vi "HSFW Engine.vi"(0 "Notifier Name":string="Not a Name", 11 "HSFW Index":string[](array[string])) -> ()   [LabVIEW 2020]
uses:
  FW Type Defs/FW Notifier Type.ctl
  FW Type Defs/FW Actions.ctl
  C:/Users/Photonics03/Documents/Microscope-Control/Device Library/Filter Wheels/Edmund Optics/HSFW 84-889/OptecHID_FilterWheelAPI.dll
  OptecHID_FilterWheelAPI.dll
panel:
  out "Current Position":u8
  in  "Get Position":bool
  in  "FW Position":u8=1 min=1 max=8
  in  "Quit":bool
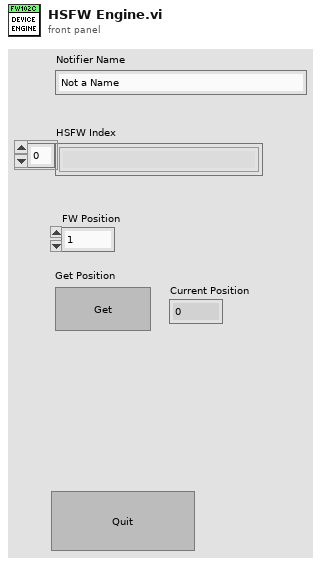
[diagram p1: front panel]
types:
  T1 = typedef "FW Actions.ctl" = enum16{"Set Position", "Get Position", "Get Num Positions", "Set Speed", "Confirm Pos", "Quit"}
  T2 = typedef "FW Notifier Type.ctl" = cluster{"Actions":T1, "Set Position":u8, "Actual Position":u8, "Speed":dbl, "Num Positions":u8, "Received":bool}
  T3 = enum32{"Invalid", "Standard", "Closed", "Hidden", "Minimized", "Maximized"}
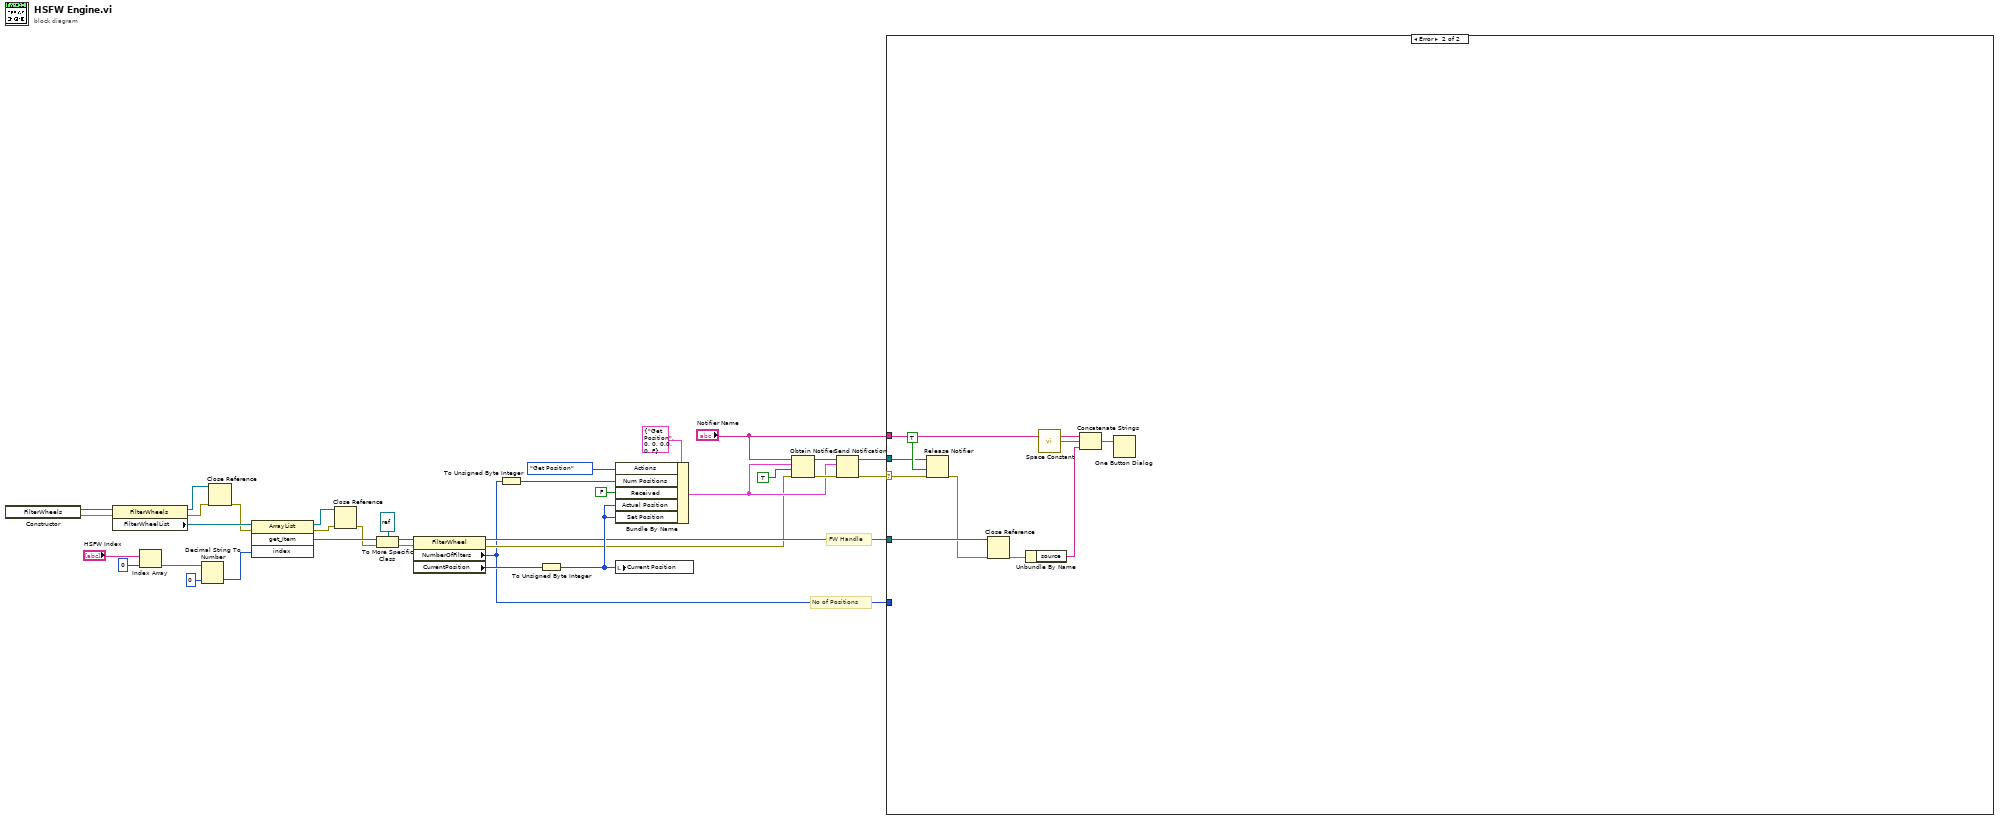
[diagram p0: block diagram]
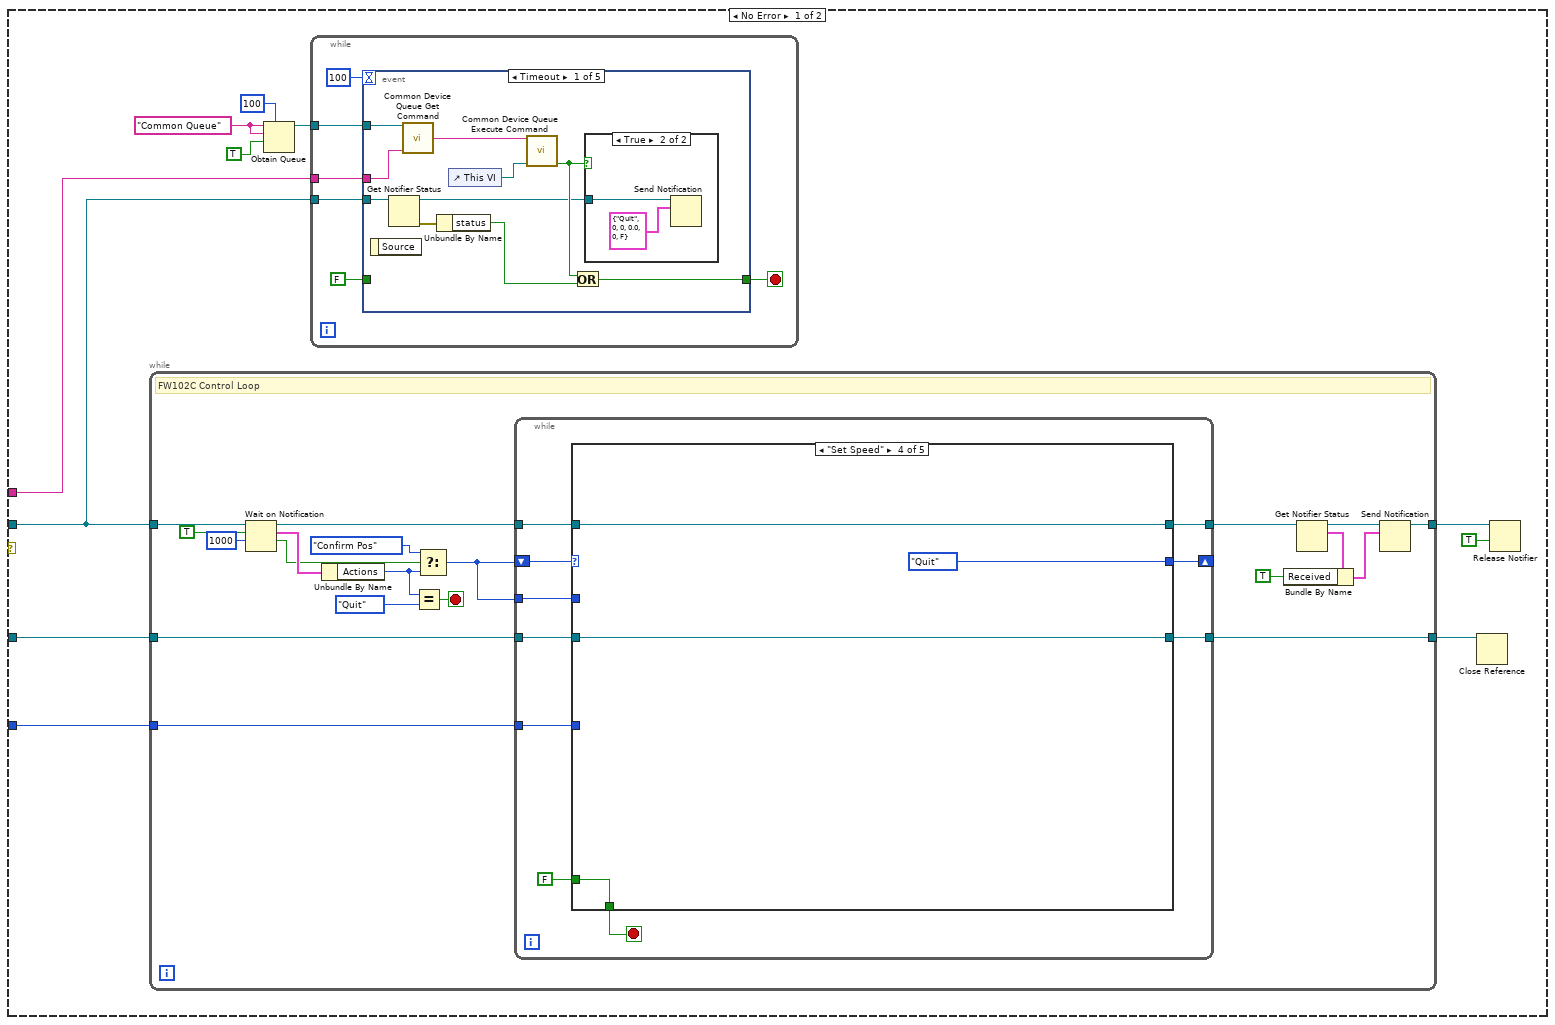
[diagram p2: hidden frame]
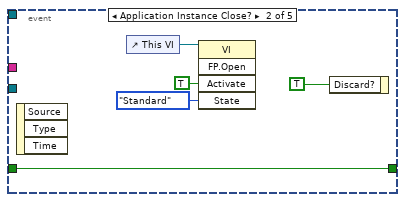
[diagram p4: hidden frame]
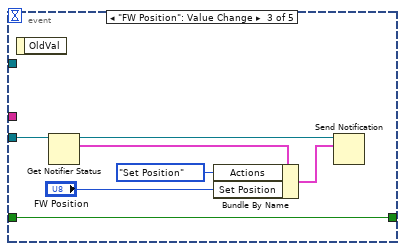
[diagram p5: hidden frame]
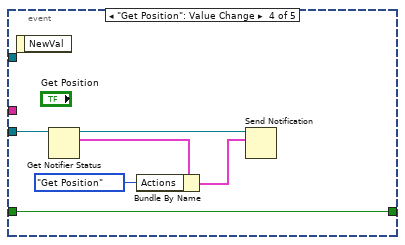
[diagram p6: hidden frame]
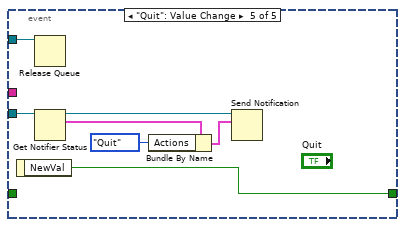
[diagram p7: hidden frame]
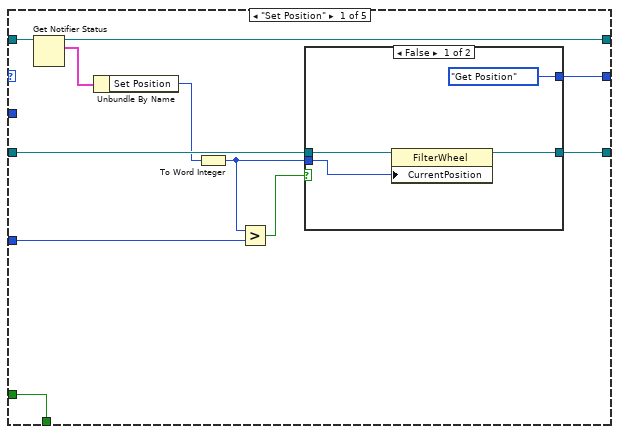
[diagram p8: hidden frame]
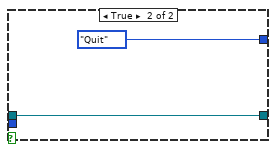
[diagram p9: hidden frame]
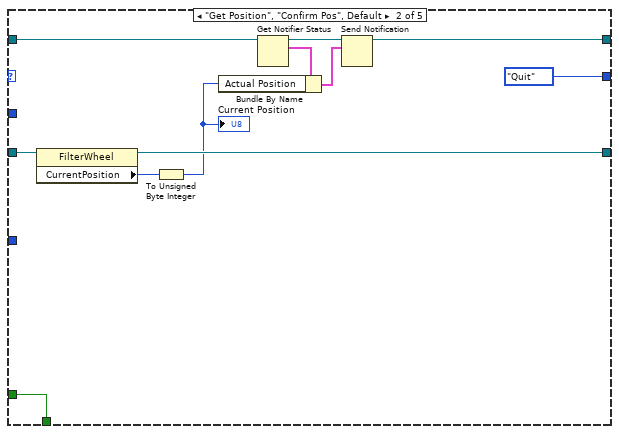
[diagram p10: hidden frame]
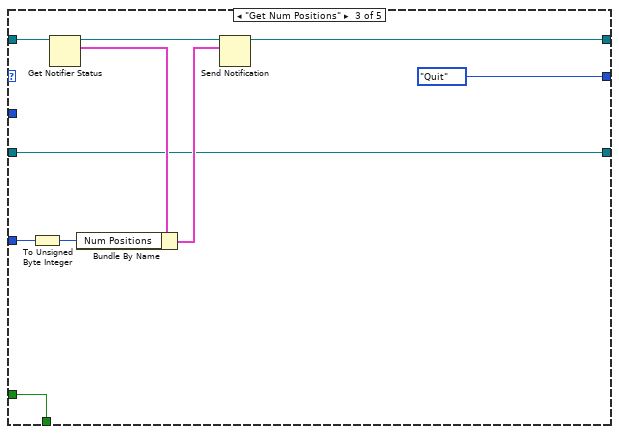
[diagram p11: hidden frame]
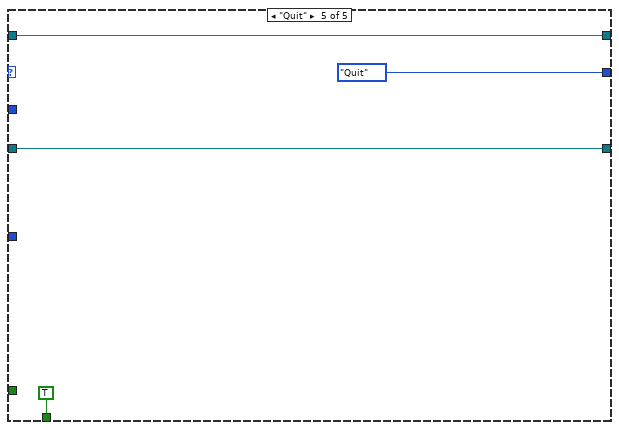
[diagram p12: hidden frame]
diagram:
  # "No of Positions"
  # "FW Handle"
  n1 = constructor class="FilterWheels"() -> (reference out=w20:refnum<k24>, error out=w17:errorcluster)  [unwired: 3 in, 1 out]
  n2 = property class="FilterWheels"(reference=w20, error in=w17) -> (reference out=w13:refnum<k24>, error out=w11:errorcluster, "FilterWheelList"=w21:refnum<k24>)
  n3 = Index Array(array="HSFW Index", index=0) -> (element=w16:string)
  n4 = Decimal String To Number(string=w16, default (0L)=0 ("default (0 I32)")) -> (number=w14:i32)  [unwired: 1 in, 1 out]
  n5 = Close Reference(reference=w13, error in (no error)=w11) -> (error out=w10:errorcluster)
  n6 = invoke class="ArrayList" method="get_Item"(reference=w21, error in=w10, "index"=w14) -> (reference out=w12:refnum<k24>, error out=w9:errorcluster, "get_Item"=w19:refnum<k24>)  [unwired: 1 in, 1 out]
  n7 = Close Reference(reference=w12, error in (no error)=w9) -> (error out=w8:errorcluster)
  n8 = To More Specific Class(target class=refnum<k24> refnum, reference=w19, error in=w8) -> (specific class reference=w7:refnum<k24>, error out=w4:errorcluster)
  n9 = property class="FilterWheel"(reference=w7, error in=w4) -> (reference out=w3:refnum<k24>, error out=w2:errorcluster, "NumberOfFilters"=w1:i16, "CurrentPosition"=w6:i16)
  n10 = To Unsigned Byte Integer(number=w1) -> (unsigned 8bit integer=w22:u8)
  n11 = To Unsigned Byte Integer(number=w6) -> (unsigned 8bit integer=w5:u8)
  n12 = Bundle By Name(cluster=T2 {"Actions"=enum."Get Position", "Set Position"=0, "Actual Position"=0, "Speed"=0.0, "Num Positions"=0, "Received"=FALSE} ("Note Type"), "Actions"=FW_Actions."Get Position", "Num Positions"=w22, "Received"=FALSE ("Received?"), "Actual Position"=w5, "Set Position"=w5) -> (w23:T2)
  n13 = local write "Current Position"(w5) -> ()
  n14 = Obtain Notifier(name (unnamed)="Notifier Name", notification data type=w23, create if not found? (T)=TRUE, error in (no error)=w2) -> (notifier out=w33:refnum<notifier>, error out=w32:errorcluster)  [unwired: 1 out]
  n15 = Send Notification(notification=w23, notifier=w33, error in (no error)=w32) -> (notifier out=w31:refnum<notifier>, error out=w30:errorcluster)
  n16 = case shown="Error" w30 {
    selector: w30 -> [_ w172]
    tunnel: w31 -> [w43 w173]
    tunnel: "Notifier Name" -> [w42 w171]
    tunnel: w3 -> [w37 w168]
    tunnel: w1 -> [w36 _]
    frame No Error {
      w41 = "Common Queue" ("Unique Notifier Name")
      n17 = while {
        tunnel: w43 -> [w102]
        tunnel: [w103] -> w44
        tunnel: w37 -> [w98]
        tunnel: [w97] -> w35
        tunnel: w36 -> [w96]
        stop <- w108 stop-if-true
        # "FW102C Control Loop"
        n18 = Wait on Notification(notifier=w102, ignore previous (F)=TRUE, timeout in ms (-1)=1000) -> (notifier out=w100:refnum<notifier>, notification=w95:T2, timed out?=w91:bool)  [unwired: 1 in, 1 out]
        n19 = Unbundle By Name(w95) -> ("Actions"=w92:T1)
        n20 = Equal?(x=w92, y=FW_Actions."Quit") -> (x = y?=w108:bool)
        n21 = Select(t=FW_Actions."Confirm Pos", s=w91, f=w92) -> (s? t:f=w90:T1)
        n22 = while {
          tunnel: w100 -> [w117]
          tunnel: [w116] -> w99
          tunnel: w98 -> [w113]
          tunnel: [w112] -> w97
          tunnel: w96 -> [w111]
          shift-right: [w110] -> _
          shift-left: w90 -> [w118]
          tunnel: w90 -> [w109]
          stop <- w114 stop-if-true
          n23 = case shown="\"Set Speed\"" w118 {
            tunnel: w117 -> [w125 w145 w155 w160 w164]
            tunnel: [w124 w143 w153 w160 w164] -> w116
            tunnel: [w129 w146 w156 w158 TRUE] -> w114
            tunnel: FALSE -> [w129 w146 w156 w158 _]
            tunnel: w113 -> [w127 w140 w147 w157 w162]
            tunnel: [w123 w138 w147 w157 w162] -> w112
            tunnel: w111 -> [w120 _ w150 _ _]
            tunnel: [w128 FW_Actions."Quit" ("f") FW_Actions."Quit" ("f") FW_Actions."Quit" ("f") FW_Actions."Quit" ("f")] -> w110
            tunnel: w109 -> [_ _ _ _ _]
            frame "Set Position" {
              n24 = Get Notifier Status(notifier=w125) -> (notifier out=w124:refnum<notifier>, current notification=w126:T2)  [unwired: 1 in, 3 out]
              n25 = Unbundle By Name(w126) -> ("Set Position"=w122:u8)
              n26 = To Word Integer(number=w122) -> (16bit integer=w121:i16)
              n27 = Greater?(x=w121, y=w120) -> (0:w119:bool)
              n28 = case shown="False" w119 {
                tunnel: [FW_Actions."Get Position" ("f") FW_Actions."Quit" ("f")] -> w128
                tunnel: w127 -> [w132 w135]
                tunnel: [w130 w135] -> w123
                tunnel: w121 -> [w131 _]
                frame False {
                  n29 = property class="FilterWheel"(reference=w132, "CurrentPosition"=w131) -> (reference out=w130:refnum<k24>)  [unwired: 1 in, 1 out]
                }
                frame True {
                }
              }
            }
            frame "Get Position", "Confirm Pos", Default {
              n30 = property class="FilterWheel"(reference=w140) -> (reference out=w138:refnum<k24>, "CurrentPosition"=w139:i16)  [unwired: 1 in, 1 out]
              n31 = To Unsigned Byte Integer(number=w139) -> (unsigned 8bit integer=w136:u8)
              "Current Position" <- w136
              n32 = Get Notifier Status(notifier=w145) -> (notifier out=w144:refnum<notifier>, current notification=w142:T2)  [unwired: 1 in, 3 out]
              n33 = Bundle By Name(cluster=w142, "Actual Position"=w136) -> (w141:T2)
              n34 = Send Notification(notification=w141, notifier=w144) -> (notifier out=w143:refnum<notifier>)  [unwired: 1 in, 1 out]
            }
            frame "Get Num Positions" {
              n35 = To Unsigned Byte Integer(number=w150) -> (unsigned 8bit integer=w149:u8)
              n36 = Get Notifier Status(notifier=w155) -> (notifier out=w154:refnum<notifier>, current notification=w151:T2)  [unwired: 1 in, 3 out]
              n37 = Bundle By Name(cluster=w151, "Num Positions"=w149) -> (w148:T2)
              n38 = Send Notification(notification=w148, notifier=w154) -> (notifier out=w153:refnum<notifier>)  [unwired: 1 in, 1 out]
            }
            frame "Set Speed" {
            }
            frame "Quit" {
            }
          }
        }
        n39 = Get Notifier Status(notifier=w99) -> (notifier out=w104:refnum<notifier>, current notification=w106:T2)  [unwired: 1 in, 3 out]
        n40 = Bundle By Name(cluster=w106, "Received"=TRUE ("Received?")) -> (w107:T2)
        n41 = Send Notification(notification=w107, notifier=w104) -> (notifier out=w103:refnum<notifier>)  [unwired: 1 in, 1 out]
      }
      n42 = Obtain Queue(max queue size (-1, unlimited)=100, name (unnamed)=w41, element data type=w41, create if not found? (T)=TRUE) -> (queue out=w38:refnum<queue>)  [unwired: 1 in, 2 out]
      n43 = while {
        tunnel: w38 -> [w51]
        tunnel: w43 -> [w48]
        tunnel: w42 -> [w46]
        stop <- w47 stop-if-true
        n44 = event shown="[0] Timeout" {
          selector: _ -> [_ _ _ _ _]
          dyn-events: _ -> [_ _ _ _ _]
          timeout: 100 -> [_ _ _ _ _]
          tunnel: w51 -> [w59 _ _ _ w84]
          tunnel: FALSE -> [_ w68 w75 w81 _]
          tunnel: w48 -> [w61 _ w74 w80 w85]
          tunnel: [w54 w68 w75 w81 w88] -> w47
          tunnel: w46 -> [w58 _ _ _ _]
          event Timeout {
            n45 = event-data() -> ()  [unwired: 1 in, 1 out]
            n46 = Get Notifier Status(notifier=w61) -> (notifier out=w52:refnum<notifier>, error out=w60:errorcluster)  [unwired: 1 in, 3 out]
            n47 = call "Common Device Queue Get Command.vi"("Common Queue"=w59, "Notifier Name"=w58) -> ("Command"=w57:string)  [unwired: 12 in, 1 out]
            n48 = Unbundle By Name(w60) -> ("status"=w55:bool)
            n49 = control-ref of="This VI"() -> (w56:refnum<vi>)
            n50 = call "Common Device Queue Execute Command.vi"("Common Command"=w57, "VI Refnum"=w56) -> ("Quit?"=w53:bool)  [unwired: 12 in, 1 out]
            n51 = Or(x=w53, y=w55) -> (x .or. y?=w54:bool)
            n52 = case shown="True" w53 {
              tunnel: w52 -> [_ w63]
              frame False {
              }
              frame True {
                n53 = Send Notification(notification=T2 {"Actions"=enum."Quit", "Set Position"=0, "Actual Position"=0, "Speed"=0.0, "Num Positions"=0, "Received"=FALSE} ("Note Type"), notifier=w63) -> ()  [unwired: 1 in, 2 out]
              }
            }
          }
          event Application Instance Close? {
            n54 = event-data() -> ()  [unwired: 1 in, 3 out]
            n55 = control-ref of="This VI"() -> (w65:refnum<vi>)
            n56 = invoke class="VI" method="FP.Open"(reference=w65, "Activate"=TRUE ("Activate?"), "State"=T3."Standard") -> ()  [unwired: 2 in, 5 out]
            n57 = event-data("Discard?"=TRUE) -> ()  [unwired: 1 in, 1 out]
          }
          event "FW Position": Value Change {
            n58 = event-data() -> ()  [unwired: 1 in, 1 out]
            n59 = Get Notifier Status(notifier=w74) -> (notifier out=w73:refnum<notifier>, current notification=w72:T2)  [unwired: 1 in, 3 out]
            n60 = Bundle By Name(cluster=w72, "Actions"=FW_Actions."Set Position", "Set Position"="FW Position") -> (w71:T2)
            n61 = Send Notification(notification=w71, notifier=w73) -> ()  [unwired: 1 in, 2 out]
          }
          event "Get Position": Value Change {
            n62 = event-data() -> ()  [unwired: 1 in, 1 out]
            n63 = Get Notifier Status(notifier=w80) -> (notifier out=w79:refnum<notifier>, current notification=w78:T2)  [unwired: 1 in, 3 out]
            n64 = Bundle By Name(cluster=w78, "Actions"=FW_Actions."Get Position") -> (w77:T2)
            n65 = Send Notification(notification=w77, notifier=w79) -> ()  [unwired: 1 in, 2 out]
          }
          event "Quit": Value Change {
            n66 = event-data() -> ("NewVal"=w88:bool)  [unwired: 1 in]
            n67 = Release Queue(queue=w84) -> ()  [unwired: 2 in, 3 out]
            n68 = Get Notifier Status(notifier=w85) -> (notifier out=w87:refnum<notifier>, current notification=w83:T2)  [unwired: 1 in, 3 out]
            n69 = Bundle By Name(cluster=w83, "Actions"=FW_Actions."Quit") -> (w86:T2)
            n70 = Send Notification(notification=w86, notifier=w87) -> ()  [unwired: 1 in, 2 out]
          }
        }
      }
      n71 = Close Reference(reference=w35) -> ()  [unwired: 1 in, 1 out]
      n72 = Release Notifier(notifier=w44, force destroy? (F)=TRUE) -> ()  [unwired: 1 in, 3 out]
    }
    frame Error {
      n73 = Release Notifier(notifier=w173, force destroy? (F)=TRUE, error in (no error)=w172) -> (error out=w167:errorcluster)  [unwired: 2 out]
      n74 = Close Reference(reference=w168, error in (no error)=w167) -> (error out=w166:errorcluster)
      n75 = Unbundle By Name(w166) -> ("source"=w165:string)
      n76 = call <vilib>:"Space Constant.vi"() -> ("String"=w169:string)
      n77 = Concatenate Strings(w171, w169, w165) -> (w170:string)
      n78 = One Button Dialog(message=w170) -> ()  [unwired: 1 in, 1 out]
    }
  }
